vi "VG_Valide.vi"() -> ()   [LabVIEW 2020]
panel:
  out "Validé?":bool
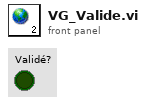
[diagram p1: front panel]
diagram:
